vi "TIME-秒.vi"   [LabVIEW 2013]
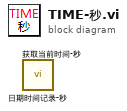
[diagram p0: block diagram]
diagram:
  n1 = call "日期时间记录-秒.vi"() -> ()  [unwired: 11 in, 1 out]
  n2 = call "获取当前时间-秒.vi"() -> ()  [unwired: 11 in, 1 out]
